vi "diffraction_rec_vi.vi"() -> ()   [LabVIEW 2017]
doc: "范例演示了使用FFT VI计算二维FFT，在原始二维图像中使用一个简单的矩形阶梯函数。范例还带有其他类型的输入，用于演示其对二维图像的影响。"
uses:
  <vilib>/Analysis/baseanly.llb/Real Outer Product.vi
  <vilib>/Analysis/2dsp.llb/2D Real FFT.vi
  <vilib>/Analysis/1siggen.llb/General Aperiodic Triangle.vi
  <vilib>/Analysis/1siggen.llb/General Gaussian Monopulse.vi
  <vilib>/Analysis/NI_AALPro.lvlib
  <vilib>/Analysis/NI_AALBase.lvlib
panel:
  in  "不对称x":dbl(slide)=0.5 step=0.1 scale=0.0..1.0
  in  "不对称y":dbl(slide)=0.5 step=0.1 scale=0.0..1.0
  in  "移位？":bool=TRUE
  in  "停止":bool
  in  "狭缝图样类型":u16(ring) items=["脉冲", "三角", "噪声", "正弦"]
  in  "狭缝透过率":dbl(slide)=100.0 scale=0.0..200.0
  out "衍射图样":dbl[][](graph)
  out "狭缝图样":dbl[][](graph)
  # "仿真了各种类型狭缝的衍射图样（远场夫琅禾费衍射）\nby 16171048 秦昊烨"
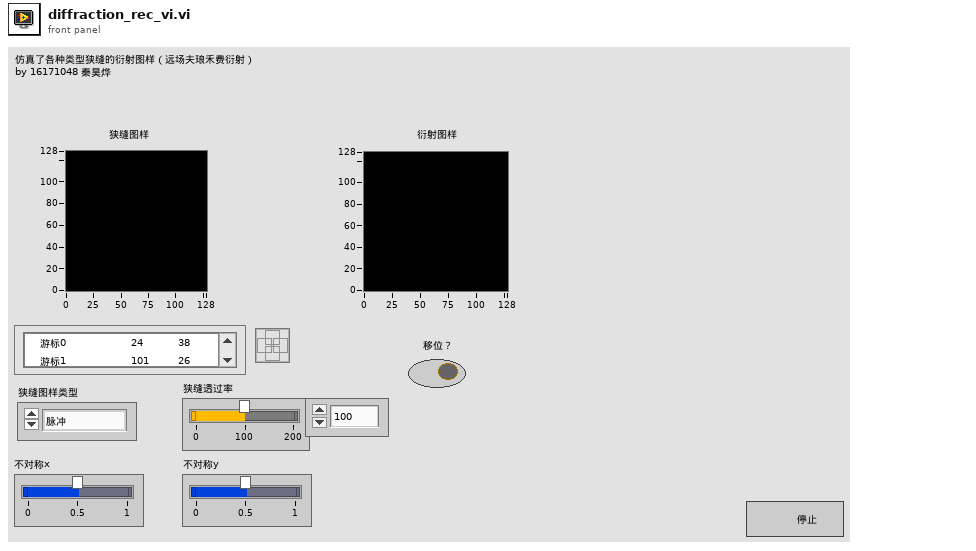
[diagram p1: front panel]
types:
  T1 = typedef "NI_Matrix.lvlib/RealMatrix.ctl" = dbl[][]
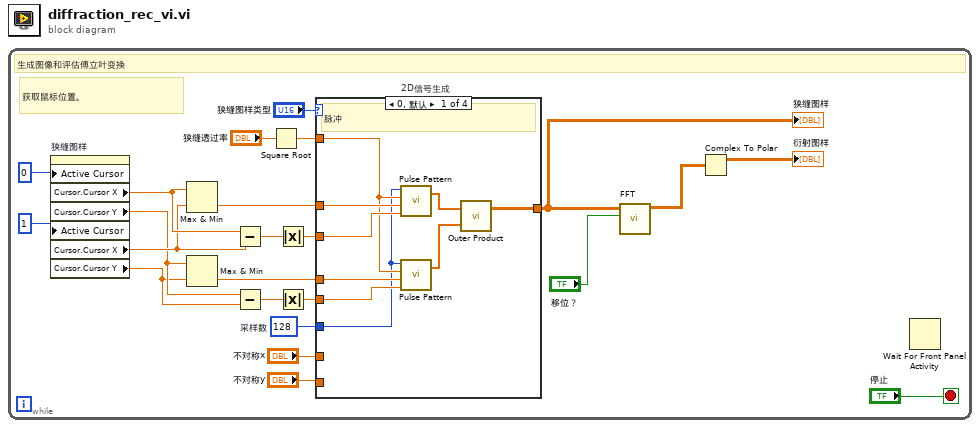
[diagram p0: block diagram]
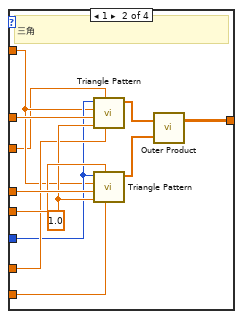
[diagram p2: hidden frame]
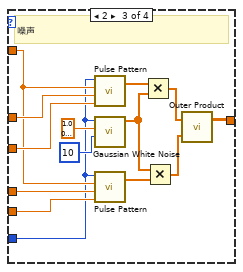
[diagram p3: hidden frame]
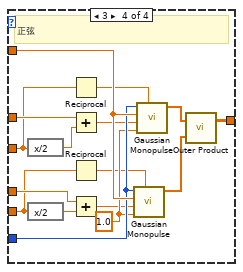
[diagram p4: hidden frame]
diagram:
  n1 = while {
    stop <- "停止" stop-if-true
    w2 = 128  # 采样数
    # "获取鼠标位置。"
    # "生成图像和评估傅立叶变换"
    n2 = property on="狭缝图样" class="IntGraph (严格)"("Active Cursor"=u32 0, "Active Cursor"=u32 1) -> ("Cursor.Cursor X"=w15:dbl, "Cursor.Cursor Y"=w10:dbl, "Cursor.Cursor X"=w14:dbl, "Cursor.Cursor Y"=w9:dbl)  [unwired: 2 in, 2 out]
    n3 = Max & Min(x=w15, y=w14) -> (min(x,y)=w17:dbl)  [unwired: 1 out]
    n4 = Max & Min(x=w10, y=w9) -> (min(x,y)=w16:dbl)  [unwired: 1 out]
    n5 = Subtract(x=w15, y=w14) -> (x-y=w13:dbl)
    n6 = Subtract(x=w10, y=w9) -> (x-y=w11:dbl)
    n7 = Square Root(x="狭缝透过率") -> (sqrt(x)=w1:dbl)
    n8 = Absolute Value(x=w13) -> (abs(x)=w12:dbl)
    n9 = Absolute Value(x=w11) -> (abs(x)=w8:dbl)
    n10 = case "2D信号生成" shown="0, 默认" "狭缝图样类型" {
      tunnel: [w30 w44 w56 w72] -> w23
      tunnel: w17 -> [w29 w43 w55 w68]
      tunnel: w12 -> [w28 w33 w54 w61]
      tunnel: w16 -> [w27 w42 w53 w66]
      tunnel: w8 -> [w26 w41 w52 w59]
      tunnel: w1 -> [w25 w36 w51 w71]
      tunnel: "不对称y" -> [_ w39 _ _]
      tunnel: "不对称x" -> [_ w38 _ _]
      tunnel: w2 -> [w24 w37 w45 w70]
      frame 0, Default {
        # "脉冲"
        n11 = call <vilib>:"Pulse Pattern.vi"("width"=w28, "delay"=w29, "amplitude"=w25, "samples"=w24) -> ("Pulse Pattern"=w32:dbl[])  [unwired: 1 out]
        n12 = call <vilib>:"Pulse Pattern.vi"("width"=w26, "delay"=w27, "amplitude"=w25, "samples"=w24) -> ("Pulse Pattern"=w31:dbl[])  [unwired: 1 out]
        n13 = call-poly <vilib>:"Outer Product.vi"("Y Vector"=w31, "X Vector"=w32) -> ("Outer Product"=w30:T1)  [unwired: 1 out]
      }
      frame 1 {
        w40 = 1.0 ("delta t (s)")
        # "三角"
        n14 = call <vilib>:"Triangle Pattern.vi"("asymmetry"=w38, "width (s)"=w33, "delta t (s)"=w40, "delay (s)"=w43, "amplitude"=w36, "samples"=w37) -> ("Triangle Pattern"=w34:dbl[])  [unwired: 4 in, 1 out]
        n15 = call <vilib>:"Triangle Pattern.vi"("asymmetry"=w39, "width (s)"=w41, "delta t (s)"=w40, "delay (s)"=w42, "amplitude"=w36, "samples"=w37) -> ("Triangle Pattern"=w35:dbl[])  [unwired: 4 in, 1 out]
        n16 = call-poly <vilib>:"Outer Product.vi"("Y Vector"=w35, "X Vector"=w34) -> ("Outer Product"=w44:T1)  [unwired: 1 out]
      }
      frame 2 {
        # "噪声"
        n17 = call <vilib>:"Pulse Pattern.vi"("width"=w54, "delay"=w55, "amplitude"=w51, "samples"=w45) -> ("Pulse Pattern"=w58:dbl[])  [unwired: 1 out]
        n18 = call <vilib>:"Gaussian White Noise.vi"("seed"=10, "standard deviation"=1.0000000000000002, "samples"=w45) -> ("Gaussian noise pattern"=w47:dbl[])  [unwired: 7 in, 1 out]
        n19 = call <vilib>:"Pulse Pattern.vi"("width"=w52, "delay"=w53, "amplitude"=w51, "samples"=w45) -> ("Pulse Pattern"=w57:dbl[])  [unwired: 1 out]
        n20 = Multiply(x=w58, y=w47) -> (x*y=w50:dbl[])
        n21 = Multiply(x=w47, y=w57) -> (x*y=w48:dbl[])
        n22 = call-poly <vilib>:"Outer Product.vi"("Y Vector"=w48, "X Vector"=w50) -> ("Outer Product"=w56:T1)  [unwired: 1 out]
      }
      frame 3 {
        w69 = 1.0 ("delta t (s)")
        # "正弦"
        n23 = expression code="x/2"(w61) -> (w62:dbl)
        n24 = expression code="x/2"(w59) -> (w64:dbl)
        n25 = Reciprocal(x=w61) -> (1/x=w63:dbl)
        n26 = Add(x=w68, y=w62) -> (x+y=w67:dbl)
        n27 = Reciprocal(x=w59) -> (1/x=w60:dbl)
        n28 = Add(x=w66, y=w64) -> (x+y=w65:dbl)
        n29 = call <vilib>:"Gaussian Monopulse.vi"("center frequency (Hz)"=w60, "delta t (s)"=w69, "delay (s)"=w65, "amplitude"=w71, "samples"=w70) -> ("Gaussian Monopulse"=w73:dbl[])  [unwired: 5 in, 1 out]
        n30 = call <vilib>:"Gaussian Monopulse.vi"("center frequency (Hz)"=w63, "delta t (s)"=w69, "delay (s)"=w67, "amplitude"=w71, "samples"=w70) -> ("Gaussian Monopulse"=w74:dbl[])  [unwired: 5 in, 1 out]
        n31 = call-poly <vilib>:"Outer Product.vi"("Y Vector"=w73, "X Vector"=w74) -> ("Outer Product"=w72:T1)  [unwired: 1 out]
      }
    }
    "狭缝图样" <- w23
    n32 = call-poly <vilib>:"FFT.vi"("shift?"="移位？", "X"=w23) -> ("FFT {X}"=w6:cdb[][])  [unwired: 8 in, 1 out]
    n33 = Complex To Polar(r * e^(i*theta)=w6) -> (r=→"衍射图样":dbl[][])  [unwired: 1 out]
    n34 = Wait For Front Panel Activity() -> ()  [unwired: 3 in, 1 out]
  }
